vi "New.vi"(5 "Abort Wait Reference 2":refnum<vi>, 7 "Abort Wait Reference":refnum<vi>, 8 "error in (no error)":errorcluster, 9 "Wait for Configuration Total Time [ms]":i32=5000, 10 "Wait for Configuration Timeout [ms]":i32=5000, 11 "Connection Settings":T1={"IP-address"="150.106.171.173", "Port"="5011", "ID Code"=1001}) -> (0 "error out":errorcluster, 3 "Statnett C37.118 DLL out":refnum<class "Statnett C37.118 DLL.lvclass">)   [LabVIEW 2013, in "PMU Recorder Light.lvlib" / "Statnett C37.118 DLL.lvclass"]
uses:
  Statnett C37.118 DLL.lvclass
  Statnett C37.118 DLL.lvclass/Statnett C37.118 DLL.ctl
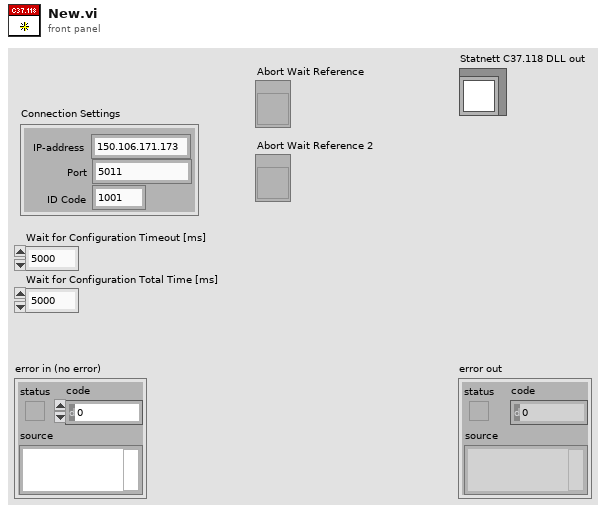
[diagram p1: front panel]
types:
  T1 = cluster{"IP-address":string, "Port":string, "ID Code":u32}
  T2 = cluster{"Time Stamp":timestamp, "Action":string, "Executed":bool, "OK":bool, "Result":string}[]
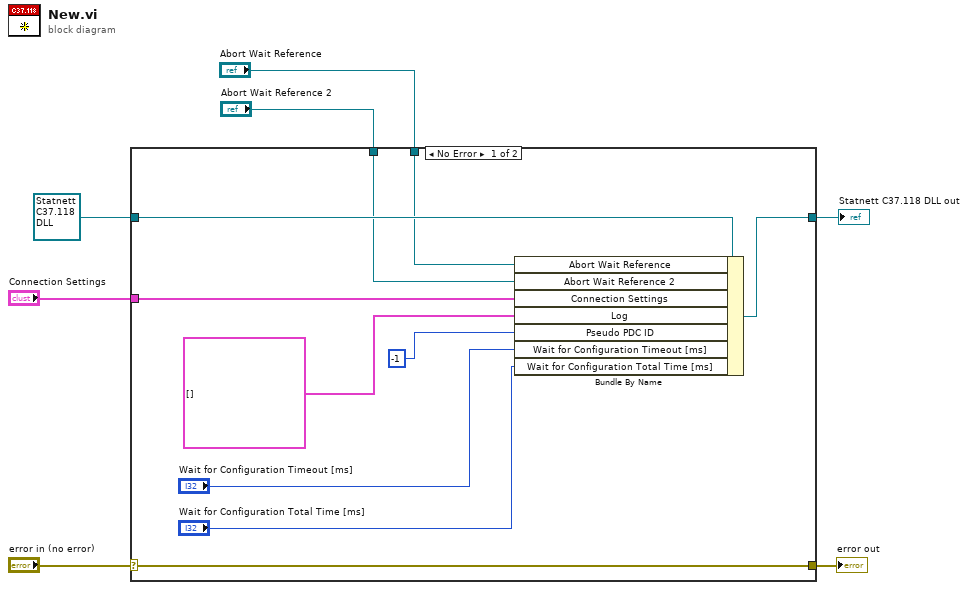
[diagram p0: block diagram]
diagram:
  n1 = case shown="No Error" "error in (no error)" {
    selector: "error in (no error)" -> [w17 w19]
    tunnel: [w17 w19] -> w6
    tunnel: [w14 w18] -> w5
    tunnel: refnum<class "Statnett C37.118 DLL.lvclass"> refnum ("Statnett C37.118 DLL in") -> [w15 w18]
    tunnel: "Connection Settings" -> [w16 _]
    tunnel: "Abort Wait Reference" -> [w9 _]
    tunnel: "Abort Wait Reference 2" -> [w8 _]
    frame No Error {
      n2 = Bundle By Name(cluster=w15, "Abort Wait Reference"=w9, "Abort Wait Reference 2"=w8, "Connection Settings"=w16, "Log"=T2 [], "Pseudo PDC ID"=-1, "Wait for Configuration Timeout [ms]"="Wait for Configuration Timeout [ms]", "Wait for Configuration Total Time [ms]"="Wait for Configuration Total Time [ms]") -> (w14:refnum<class "Statnett C37.118 DLL.lvclass">)
    }
    frame Error {
    }
  }
  "error out" <- w6
  "Statnett C37.118 DLL out" <- w5
